vi "CODcr全局变量.vi"() -> ()   [LabVIEW 2016, in "CODCr库.lvlib"]
uses:
  <vilib>/Plasmionique/MB Master/MB_Master_Serial/MB_Master_Serial.lvclass
panel:
  in  "Error in":errorcluster
  in  "MB_Serial session":refnum<class "MB_Master_Serial.lvclass">
  in  "VISA Resource":refnum<visa-resource-name>="COM9"
  out "工作状态":T1(ring)
  out "测量状态":string
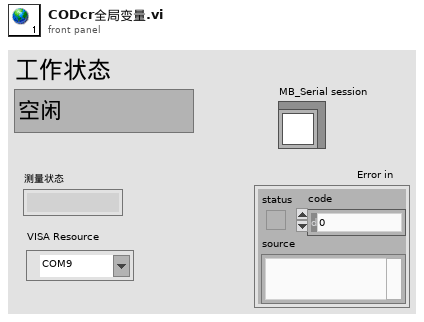
[diagram p1: front panel]
types:
  T1 = enum16{"空闲", "水样测试", "标样核查", "零点核查", "跨度核查", "空白测试", "平行样测试", "加标回收", "空白校准", "标样校准", "初始化（清洗）"}
diagram:
